vi "Pneumatic Read.vi"() -> (0 "Shooter":dbl, 1 "Line":dbl)   [LabVIEW 2013]
uses:
  Robot Global Data.vi
  <vilib>/addons/control/pid/pid.llb/PID Control Input Filter (DBL).vi
  <vilib>/addons/control/pid/NI_PID_pid.lvlib
panel:
  out "Line":dbl(graph)
  out "Shooter":dbl(graph)
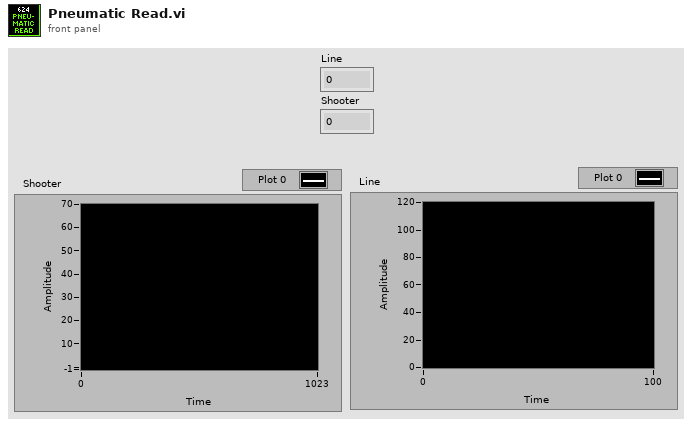
[diagram p1: front panel]
types:
  T1 = typedef "Dashboard UDP Packet.ctl" = cluster{"Camera":T2, "Gyro":T3, "Encoder":T5, "Auto Shift":T6, "Auton":T7, "Drive/Ramp X":dbl, "Drive/Ramp Y":dbl, "Drive/Battery Cutoff":dbl, "Pressure/Compressor Min Voltage":dbl, "Pressure/Compressor Delay":dbl, "Controller/Strafe Correction":bool, "Shooter":T8, "Rollers":T9, "Abort":bool, "Finish":bool}
  T2 = typedef "Camera Controls.ctl" = cluster{"Camera/View Angle X":dbl, "Camera/Goal Track Timeout":dbl, "Camera/View Angle Y":dbl, "Camera/Goal Exposure":dbl, "Camera/Vision Receive Timeout":dbl, "Camera/Offset 1":dbl, "Camera/Offset 2":dbl}
  T3 = typedef "Gyro Controls.ctl" = cluster{"Gyro/Angle Tolerance":dbl, "Gyro/Steer Closeness Threshold":dbl, "Steer PID":T4, "Steer Close PID":T4}
  T4 = typedef "PID Params.ctl" = cluster{"max":dbl, "min":dbl, "P":dbl, "I":dbl, "D":dbl}
  T5 = typedef "Encoder Controls.ctl" = cluster{"Encoders/Reset":bool, "Encoders/Omni Constant":dbl, "Encoders/Omni Tick Constant":dbl, "Encoders/Left Constant":dbl, "Encoders/Right Constant":dbl, "Encoders/Right Tick Constant":dbl}
  T6 = typedef "Auto Shift Controls.ctl" = cluster{"AutoShift/Upshift Throttle Accel":dbl, "AutoShift/Speed Threshold":dbl, "AutoShift/Upshift Throttle":dbl, "AutoShift/Upshift Accel":dbl, "AutoShift/Downshift Accel":dbl, "AutoShift/Downshift Throttle":dbl, "AutoShift/Delay":dbl, "AutoShift/Enabled":bool}
  T7 = typedef "Auton Controls.ctl" = cluster{"Auton/Left Shoot X-Coord":dbl, "Auton/Right Shoot X-Coord":dbl, "DistDrive/Distance Stop Threshold":dbl, "DistDrive/Max Stop Speed":dbl, "Auton/Back Piston Time":dbl, "Auton/Manual Hot":bool, "Auton/Manual Hot Right":bool, "Default X PID":T4, "Default Y PID":T4}
  T8 = typedef "Shooter Controls.ctl" = cluster{"Shooter/Reset Time":dbl, "Shooter/Release Delay":dbl, "Shooter/Pressure Steady Time":dbl, "Shooter/Misfire Delay":dbl, "Shooter/Ball Settle Time":dbl, "Shooter/Line IR Delay":dbl, "Pressure/Upper PSI Time":dbl, "Pressure/Lower PSI Time":dbl, "Shooter/Punch Delay":dbl, "Shooter/Target Pressure":dbl, "Pressure/Line B":dbl, "Pressure/Line M":dbl, "Pressure/Shooter M":dbl, "Pressure/Shooter B":dbl}
  T9 = typedef "Roller Controls.ctl" = cluster{"Roller/Load IRs Verify Time":dbl, "Roller/Center IR Latch Time":dbl, "Roller/Speed Front":dbl, "Roller/Speed Back":dbl, "Roller/Entry Timeout":dbl, "Roller/To Center Timeout":dbl, "Roller/Sustain Time":dbl, "Roller/Verify Center Time":dbl}
  T10 = typedef "WPI_AnalogChannelDevRef.ctl" = cluster{"DevStatus":errorcluster, "Analog Module":T11, "Analog Channel":T12}
  T11 = typedef "FPGA_TypedefAnalogModule.ctl" = enum16{"Analog Module 1", "Analog Module 2"}
  T12 = typedef "FPGA_AIChannel.ctl" = enum8{"AI 1", "AI 2", "AI 3", "AI 4", "AI 5", "AI 6", "AI 7", "AI 8", "Invalid"}
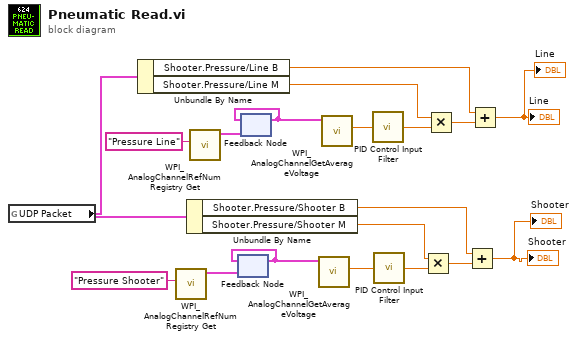
[diagram p0: block diagram]
diagram:
  n1 = global read "Robot Global Data.vi" "UDP Packet"() -> (w3:T1)
  n2 = Unbundle By Name(w3) -> ("Shooter.Pressure/Line B"=w4:dbl, "Shooter.Pressure/Line M"=w5:dbl)
  n3 = call <vilib>:"WPI_AnalogChannelRefNum Registry Get.vi"("refnum name"="Pressure Shooter") -> ("AIDeviceRef"=w12:T10)  [unwired: 9 in, 1 out]
  n4 = Unbundle By Name(w3) -> ("Shooter.Pressure/Shooter B"=w2:dbl, "Shooter.Pressure/Shooter M"=w1:dbl)
  n5 = call <vilib>:"WPI_AnalogChannelRefNum Registry Get.vi"("refnum name"="Pressure Line") -> ("AIDeviceRef"=w17:T10)  [unwired: 9 in, 1 out]
  n6 = feedback #1(w12) -> (w13:T10)
  n7 = feedback-in #1(w13) -> ()
  n8 = feedback #2(w17) -> (w16:T10)
  n9 = feedback-in #2(w16) -> ()
  n10 = call <vilib>:"WPI_AnalogChannelGetAverageVoltage.vi"("AIDeviceRef"=w13) -> ("Voltage"=w9:dbl)  [unwired: 8 in, 2 out]
  n11 = call <vilib>:"WPI_AnalogChannelGetAverageVoltage.vi"("AIDeviceRef"=w16) -> ("Voltage"=w11:dbl)  [unwired: 8 in, 2 out]
  n12 = call-poly <vilib>:"PID Control Input Filter.vi"("input"=w11) -> ("output"=w10:dbl)  [unwired: 4 in]
  n13 = call-poly <vilib>:"PID Control Input Filter.vi"("input"=w9) -> ("output"=w8:dbl)  [unwired: 4 in]
  n14 = Multiply(x=w1, y=w8) -> (x*y=w14:dbl)
  n15 = Multiply(x=w5, y=w10) -> (x*y=w15:dbl)
  n16 = Add(x=w2, y=w14) -> (x+y=→"Shooter" →"Shooter":dbl)
  n17 = Add(x=w4, y=w15) -> (x+y=→"Line" →"Line":dbl)
